vi "isSubnodeOf.vi"(8 "error in (no error)":errorcluster, 10 "subNode*":refnum<data-value>, 11 "superNode in":refnum<class "xceNode.lvclass">) -> (0 "error out":errorcluster, 2 "isSubNode":bool, 3 "superNode out":refnum<class "xceNode.lvclass">)   [LabVIEW 2013, in "xceNode.lvclass"]
doc: "Checks to see if a node is a subNode of another node."
uses:
  xceNode.lvclass
  xceTreeObj/xceTreeObj.lvclass
  xceNode.lvclass/xceNode.ctl
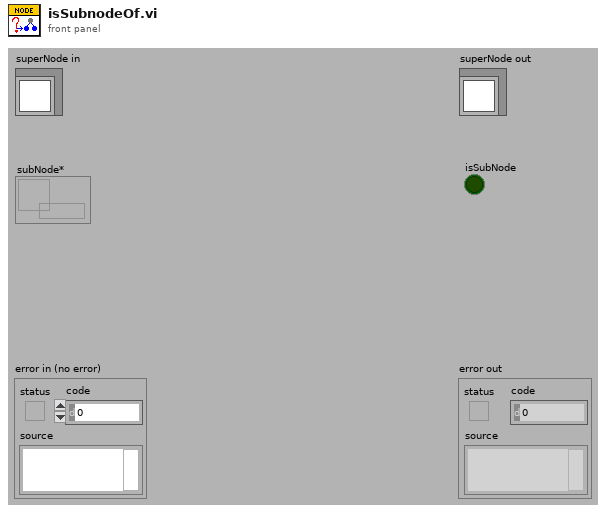
[diagram p1: front panel]
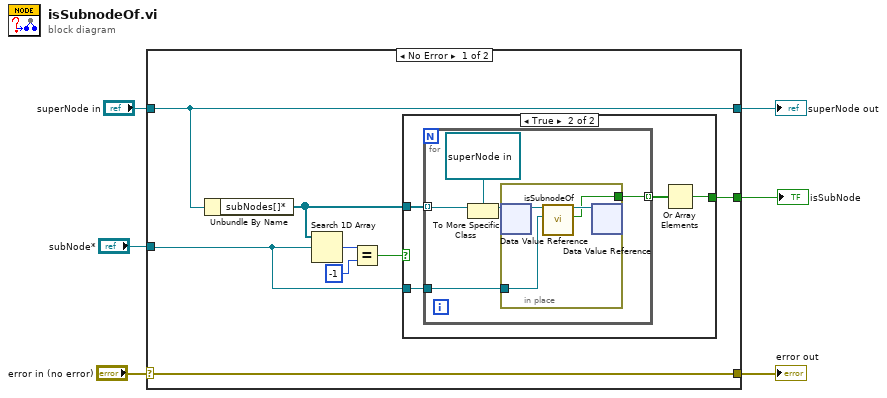
[diagram p0: block diagram]
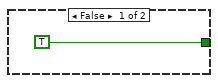
[diagram p2: hidden frame]
diagram:
  n1 = case shown="No Error" "error in (no error)" {
    selector: "error in (no error)" -> [w14 w30]
    tunnel: [w14 w30] -> w5
    tunnel: [w8 w29] -> w4
    tunnel: "superNode in" -> [w8 w29]
    tunnel: "subNode*" -> [w7 _]
    tunnel: [w10 _] -> w1
    frame No Error {
      n2 = Unbundle By Name(w8) -> ("subNodes[]*"=w9:refnum<data-value>[])
      n3 = Search 1D Array(1D array=w9, element=w7) -> (index of element=w13:i32)  [unwired: 1 in]
      n4 = Equal?(x=w13, y=-1 ("index of element")) -> (x = y?=w11:bool)
      n5 = case shown="True" w11 {
        tunnel: [TRUE w16] -> w10
        tunnel: w9 -> [_ w19]
        tunnel: w7 -> [_ w18]
        frame False {
        }
        frame True {
          n6 = for {
            tunnel: w19 -> [w24] mode=indexing
            tunnel: w18 -> [w21]
            tunnel: [w20] -> w17 mode=indexing
            n7 = To More Specific Class(target class=refnum<data-value> refnum ("data value reference"), reference=w24) -> (specific class reference=w22:refnum<data-value>)  [unwired: 1 in, 1 out]
            n8 = in-place {
              in-place-border: w21 -> [w26]
              in-place-border: [w25] -> w20
              n9 = in-place-dvr #1(w22) -> (w28:refnum<class "xceNode.lvclass">)  [unwired: 1 out]
              n10 = call "isSubnodeOf.vi"("subNode*"=w26, "superNode in"=w28) -> ("isSubNode"=w25:bool, "superNode out"=w27:refnum<class "xceNode.lvclass">)  [unwired: 7 in, 1 out]
              n11 = in-place-dvr #1(w27) -> ()  [unwired: 2 out]
            }
          }
          n12 = Or Array Elements(Boolean array=w17) -> (logical OR=w16:bool)
        }
      }
    }
    frame Error {
    }
  }
  "error out" <- w5
  "superNode out" <- w4
  "isSubNode" <- w1
